vi "Write Command (Hex).vi"(8 "error in (no error)":errorcluster, 10 "Command (Hex)":string, 11 "Hitronics in":refnum<class "Hitronics.lvclass">) -> (0 "error out":errorcluster, 3 "Hitronics out":refnum<class "Hitronics.lvclass">)   [LabVIEW 2018, in "Hitronics.lvlib" / "Hitronics.lvclass"]
uses:
  Hitronics.lvclass
  Hitronics.lvclass/Hitronics.ctl
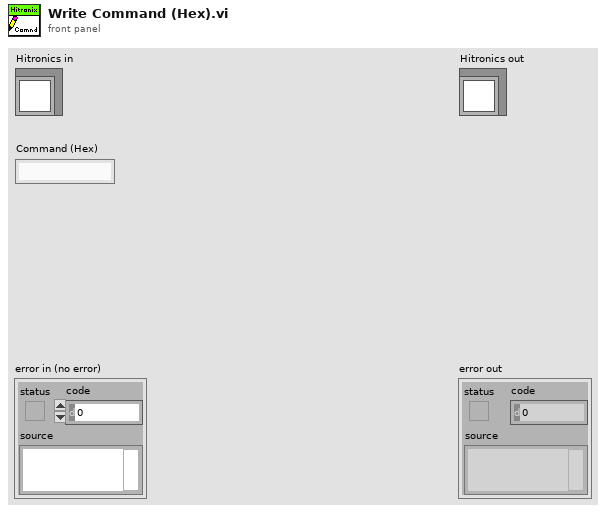
[diagram p1: front panel]
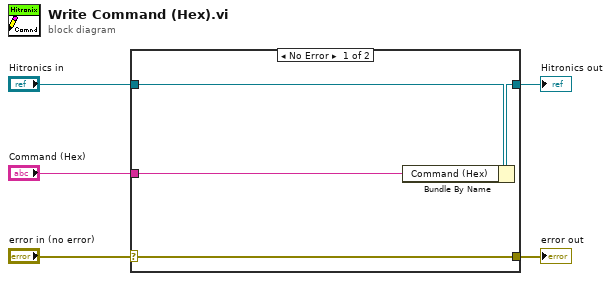
[diagram p0: block diagram]
diagram:
  n1 = case shown="No Error" "error in (no error)" {
    selector: "error in (no error)" -> [w9 w10]
    tunnel: [w9 w10] -> w4
    tunnel: [w7 w11] -> w2
    tunnel: "Hitronics in" -> [w8 w11]
    tunnel: "Command (Hex)" -> [w6 _]
    frame No Error {
      n2 = Bundle By Name(cluster=w8, "Command (Hex)"=w6) -> (w7:refnum<class "Hitronics.lvclass">)
    }
    frame Error {
    }
  }
  "error out" <- w4
  "Hitronics out" <- w2
